vi "get.vi"(7 "LabVIEW Web Service Request":refnum<class "Web Request.lvclass"> caption="LabVIEW Web服务请求") -> ()   [LabVIEW 2014]
uses:
  <vilib>/wsapi/Web Request.lvclass
panel:
  # "Web服务请求输入接线端用于调用“Web服务”选板的VI。除非不需要访问该选板，否则不要在连线板上删除这个输入接线端。"
  # "添加至连线板的每一个其他输入控件，在URL中对应于一个输入。如需在接线端模式输出（默认设置）下包含输出控件，则该输出控件必须与连线板相连。"
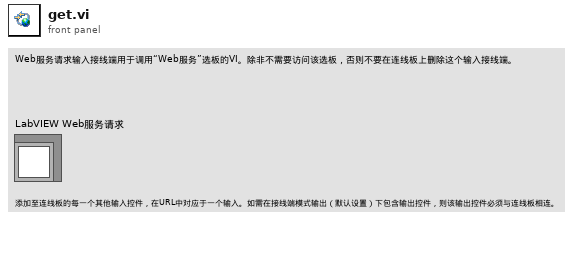
[diagram p1: front panel]
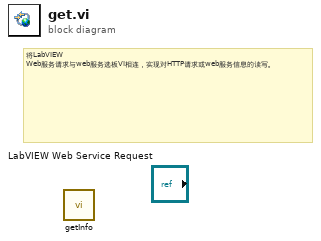
[diagram p0: block diagram]
diagram:
  # "将LabVIEW Web服务请求与web服务选板VI相连，实现对HTTP请求或web服务信息的读写。"
  n1 = call "getInfo.vi"() -> ()  [unwired: 12 in]
